vi "dscDIOSetConfig.vi"(8 "error in":errorcluster, 10 "config_bytes":u8=155 format="%x", 11 "board":i16) -> (0 "error out":errorcluster, 3 "boardOut":i16)   [LabVIEW 2011, in "Diamond Universal Driver.lvlib"]
doc: "At startup, all DIO ports are set for input. Using this VI, the user can set the direction of the different ports (the default of the control (<B>config bytes</B>) is all set for input. Refer to the manual for acceptable values."
uses:
  Diamond Universal Driver.lvlib
  Controls/error codes.ctl
  Instruments/WL OPC/Support/dlls/dscud.dll
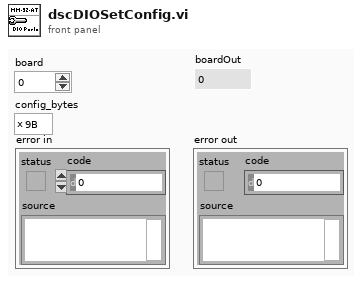
[diagram p1: front panel]
types:
  T1 = typedef "Diamond Universal Driver.lvlib/error codes.ctl" = enum8{"DE_NONE", "DE_HW_FAILURE", "DE_SW_FAILURE", "DE_HW_NOT_SUPPORTED", "DE_SW_NOT_SUPPORTED", "DE_INVALID_PARM", "DE_ALTERNATE_IN_PROGRESS", "DE_NONE_IN_PROGRESS", "DE_BUFFER_ROLLOVER", "DE_INVALID_ERROR_CODE", "DE_ALREADY_PAUSED", "DE_OVERFLOW", "DE_INVALID_FUNC", "DE_DSCUDH_INVALID", "DE_INVALID_BOARD", "DE_BOARD_LIMIT_REACHED", "DE_BOARD_BUSY", "DE_INVALID_WINDRVR_HANDLE", "DE_INVALID_WINDRVR_VERSION", "DE_BAD_WINDRVR_BOARD_INIT", "DE_OPERATION_TIMED_OUT", "DE_INVALID_WINDRVR_KP", "DE_THREAD_FAILURE"}
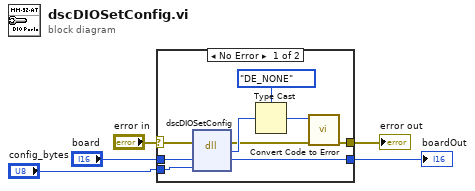
[diagram p0: block diagram]
diagram:
  n1 = case shown="No Error" "error in" {
    selector: "error in" -> [w14 w16]
    tunnel: [w10 w16] -> w4
    tunnel: [w8 w15] -> w3
    tunnel: "board" -> [w7 w15]
    tunnel: "config_bytes" -> [w6 _]
    frame No Error {
      n2 = dll-call lib="C:/Users/mrichardson/Documents/Web Based Version Control SW/Instruments/WL OPC/Support/dlls/dscud.dll" fn="dscDIOSetConfig"(error in=w14, "board"=w7, "config_bytes"=w6) -> (error out=w9:errorcluster, "error"=w13:u8, "board"=w8:i16)  [unwired: 3 in, 1 out]
      n3 = Type Cast(type=error_codes."DE_NONE" ("error codes"), x=w13) -> (*(type *) &x=w11:T1)
      n4 = call "Convert Code to Error.vi"("error in"=w9, "error codes"=w11) -> ("error out"=w10:errorcluster)  [unwired: 9 in]
    }
    frame Error {
    }
  }
  "error out" <- w4
  "boardOut" <- w3
